vi "Evaluate Continue on Failure_Do.vi"(8 "error in (no error)":errorcluster, 9 "Report":refnum<class "Report Data.lvclass">, 10 "Build Step":T1, 11 "Project Builder in":refnum<class "Project Builder.lvclass">) -> (0 "error out":errorcluster, 1 "Continue?":bool, 3 "Project Builder out":refnum<class "Project Builder.lvclass">)   [LabVIEW 2019, in "ProjectBuilder.lvlib" / "Project Builder.lvclass"]
doc: "Determines behaviour when an action fails.\n\nDefault implementation will continue through Deploy and Report but abort on all other steps."
uses:
  Project Builder.lvclass
  Ctl/Ctl_Build Steps.ctl
  ProjectBuilder.lvlib
  Data/Report Data/Report Data.lvclass
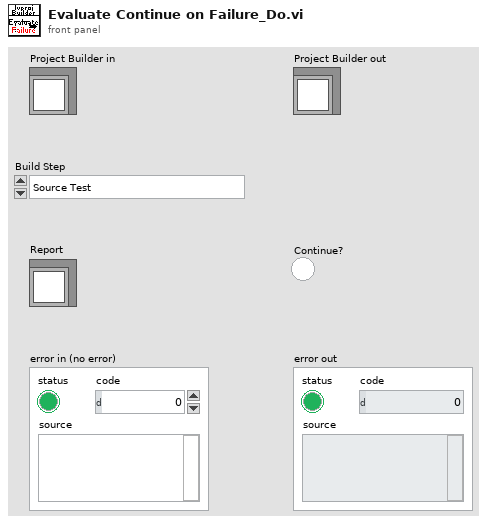
[diagram p1: front panel]
types:
  T1 = typedef "ProjectBuilder.lvlib/Ctl_Build Steps.ctl" = enum16{"Source Test", "Build", "Post-Build Test", "Deploy", "Report"}
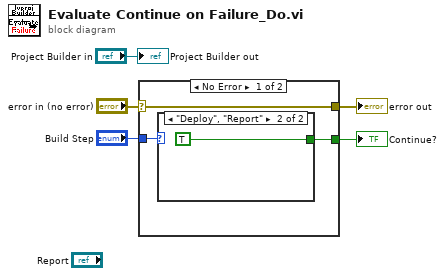
[diagram p0: block diagram]
diagram:
  n1 = case shown="No Error" "error in (no error)" {
    selector: "error in (no error)" -> [w7 w10]
    tunnel: "Build Step" -> [w8 _]
    tunnel: [w7 w10] -> w2
    tunnel: [w6 _] -> w1
    frame No Error {
      n2 = case shown="\"Deploy\", \"Report\"" w8 {
        tunnel: [_ TRUE] -> w6
        frame Default {
        }
        frame "Deploy", "Report" {
        }
      }
    }
    frame Error {
    }
  }
  "Continue?" <- w1
  "error out" <- w2
  "Project Builder out" <- "Project Builder in"
